vi "Autonomous Independent.vi"() -> ()   [LabVIEW 2013]
doc: "This VI is called when autonomous begins, and will automatically be terminated when autonomous ends. You can carry out timed or sensor driven robot movement independently without needing to return to the caller."
uses:
  Robot Global Data.vi
  OneBall.ctl
  DoubleSolenoidControl.ctl
  ShooterAction.ctl
  TwoBall.ctl
  CollectorEnum.ctl
  RollerStates.ctl
  TankDriveAction.ctl
panel:
  out "Error out 2":errorcluster
  in  "Error in 2":errorcluster
  out "Error out":errorcluster
  in  "Error in":errorcluster
  # "Be sure to right-click and choose Data Operations>>Make Current Value default if you want to save the array values with the VI"
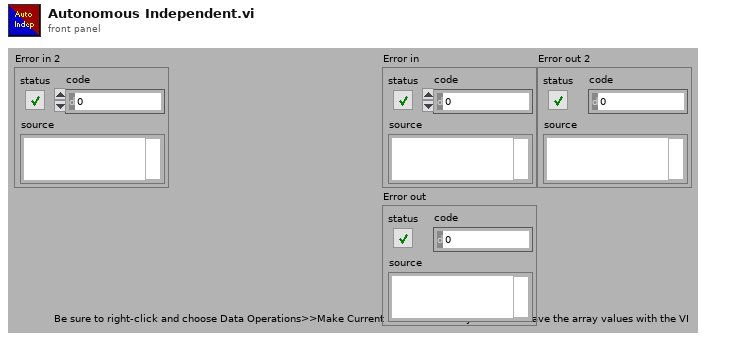
[diagram p1: front panel]
types:
  T1 = typedef "TwoBall.ctl" = enum16{"Init", "Lower Arm", "Spin Roller", "Clapper", "RaiseArmSlightly", "Drive", "Shoot1", "RaiseArmUp", "Shoot2", "Stop"}
  T2 = typedef "OneBall.ctl" = enum16{"Init", "Drive", "Shoot", "CheckGoal", "Stop"}
  T3 = typedef "WPI_JoystickDevRef.ctl" = cluster{"Device":T4}
  T4 = typedef "WPI_JoystickDeviceEnum.ctl" = enum16{"USB 1", "USB 2", "USB 3", "USB 4", "Kinect 1", "Kinect 2"}
  T5 = cluster{"axis 1 (x)":dbl, "axis 2 (y)":dbl, "axis 3 (throttle)":dbl, "axis 4":dbl, "axis 5":dbl, "axis 6":dbl}
  T6 = typedef "DoubleSolenoidControl.ctl" = enum16{"Init", "Out", "In", "Middle"}
  T7 = typedef "CollectorEnum.ctl" = enum16{"Init", "Raise", "Lower", "Stop", "GetStatus"}
  T8 = typedef "TankDriveAction.ctl" = enum16{"Init", "LinearDrive", "SetValue", "Disable"}
  T9 = typedef "RollerStates.ctl" = enum16{"Init", "Off", "Forward", "Reverse"}
  T10 = typedef "ShooterAction.ctl" = enum16{"Init", "Shoot"}
  T11 = typedef "WPI_SolenoidDevRef.ctl" = cluster{"DevStatus":errorcluster, "Solenoid Module":T12, "Forward Solenoid Channel":T13, "Reverse Solenoid Channel":T13}
  T12 = typedef "FPGA_TypedefSolenoidModule.ctl" = enum16{"Solenoid Module 1", "Solenoid Module 2"}
  T13 = typedef "WPI_SolenoidChannel.ctl" = enum8{"Solenoid 1", "Solenoid 2", "Solenoid 3", "Solenoid 4", "Solenoid 5", "Solenoid 6", "Solenoid 7", "Solenoid 8", "Invalid"}
  T14 = typedef "WPI_RelayDevRef.ctl" = cluster{"DevStatus":errorcluster, "Relay Channel":T15, "Digital Module":T16, "Relay Direction":T17}
  T15 = typedef "FPGA_DIORelayChannel.ctl" = enum8{"Relay 1", "Relay 2", "Relay 3", "Relay 4", "Relay 5", "Relay 6", "Relay 7", "Relay 8", "Invalid"}
  T16 = typedef "FPGA_TypedefDigitalModule.ctl" = enum16{"Digital Module 1", "Digital Module 2"}
  T17 = typedef "WPI_RelayDirection.ctl" = enum16{"Both directions", "Forward only", "Reverse only"}
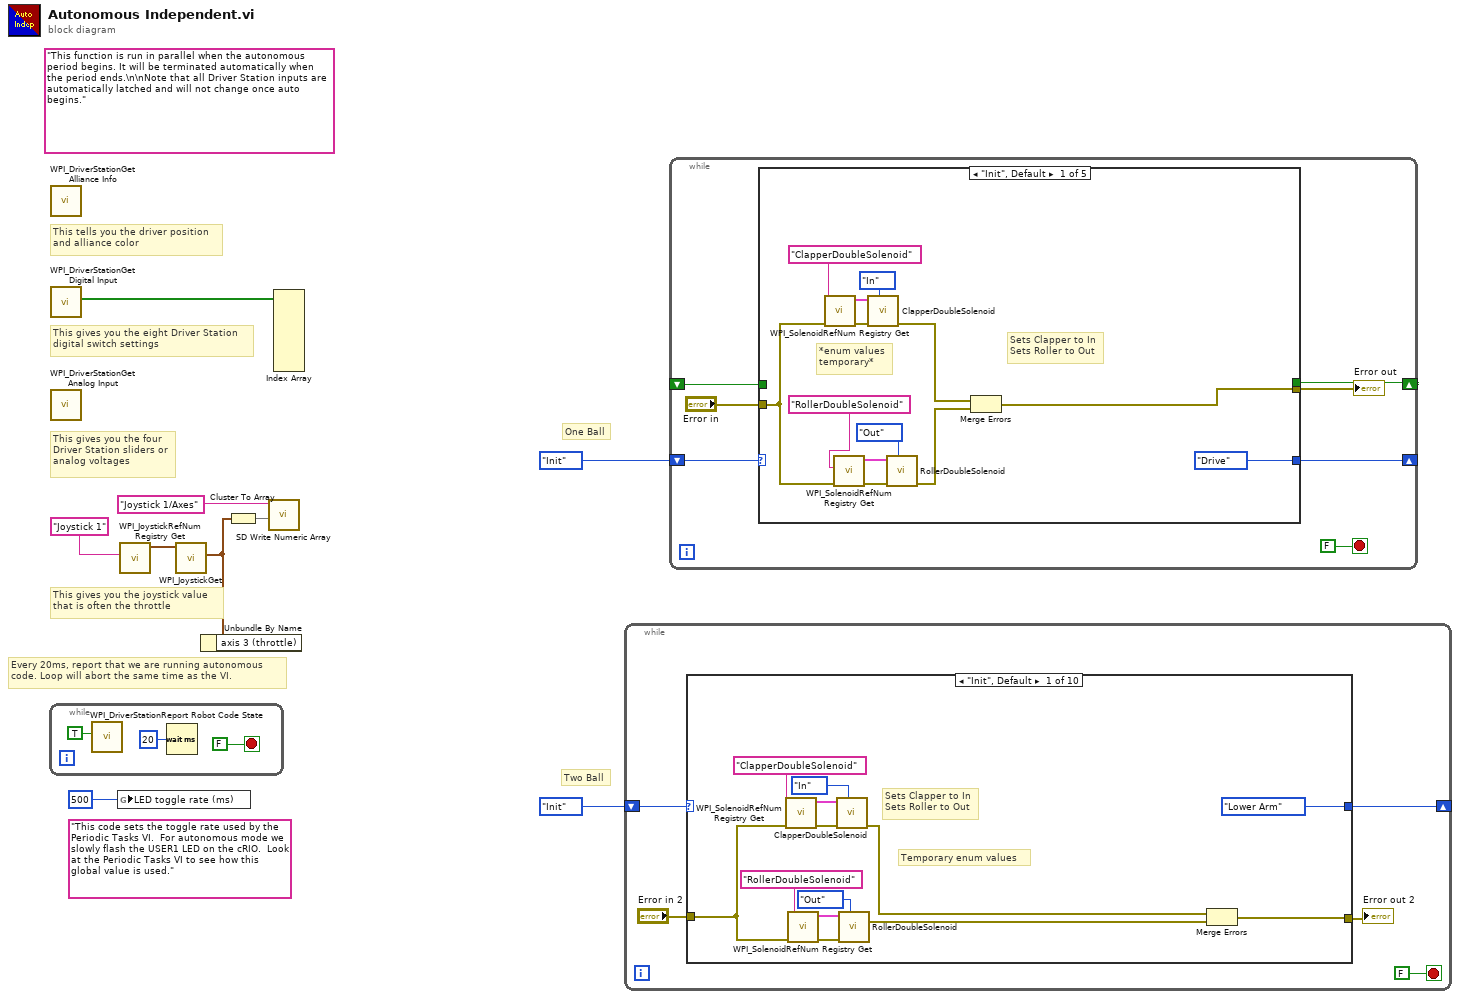
[diagram p0: block diagram]
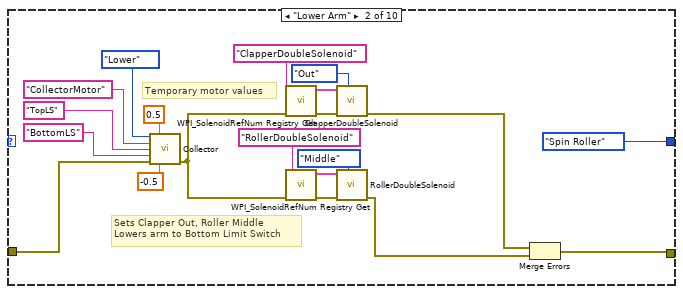
[diagram p2: hidden frame]
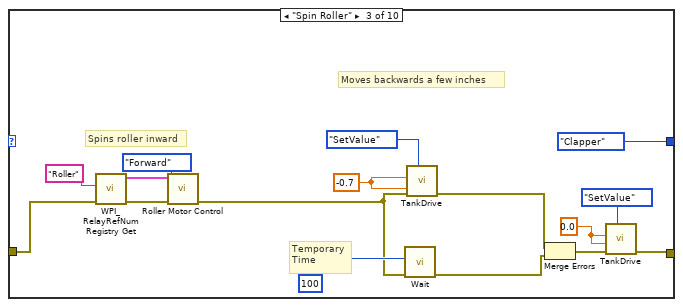
[diagram p3: hidden frame]
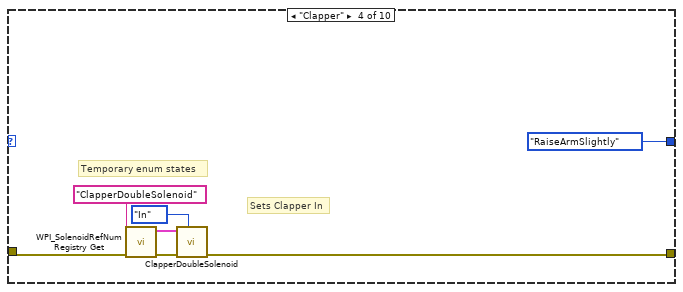
[diagram p4: hidden frame]
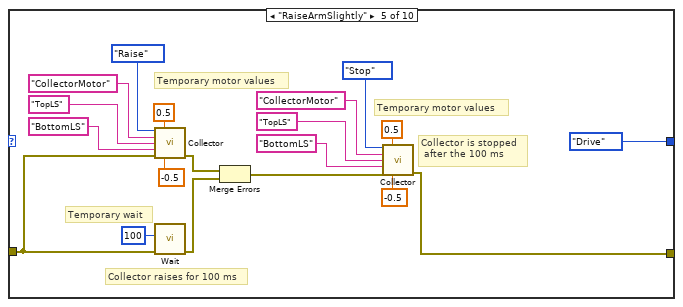
[diagram p5: hidden frame]
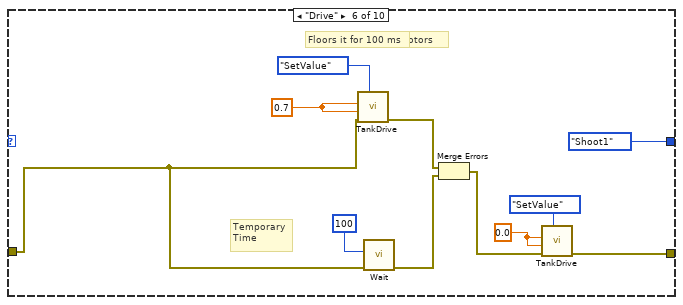
[diagram p6: hidden frame]
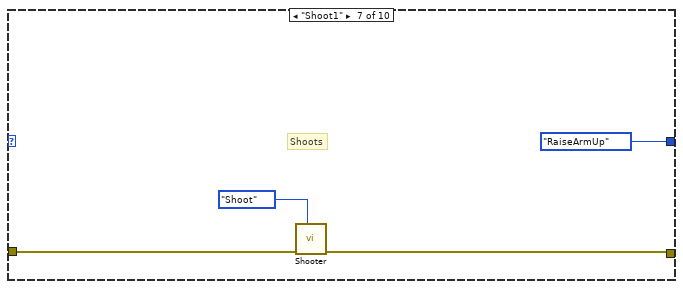
[diagram p7: hidden frame]
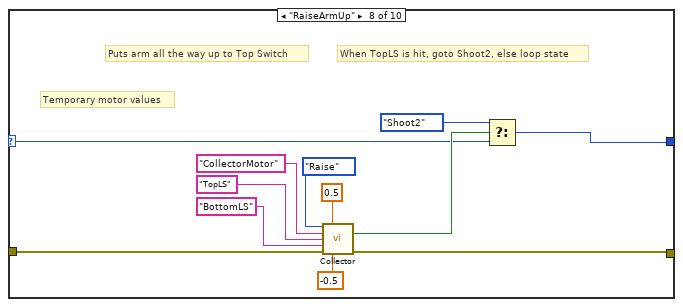
[diagram p8: hidden frame]
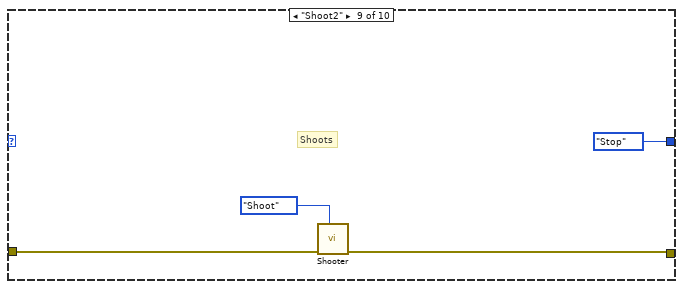
[diagram p9: hidden frame]
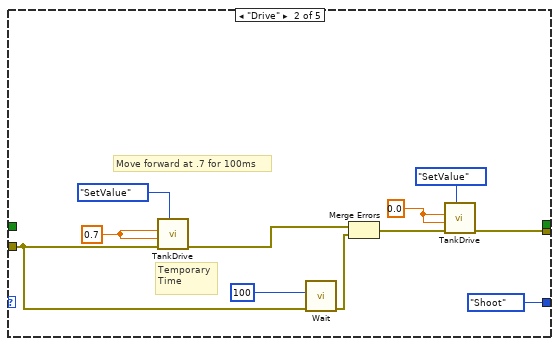
[diagram p11: hidden frame]
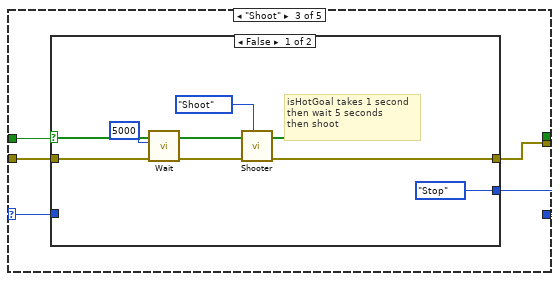
[diagram p12: hidden frame]
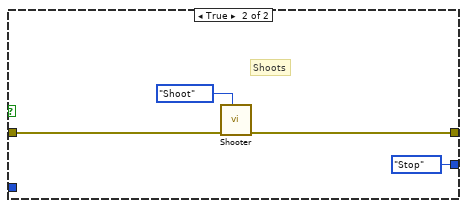
[diagram p13: hidden frame]
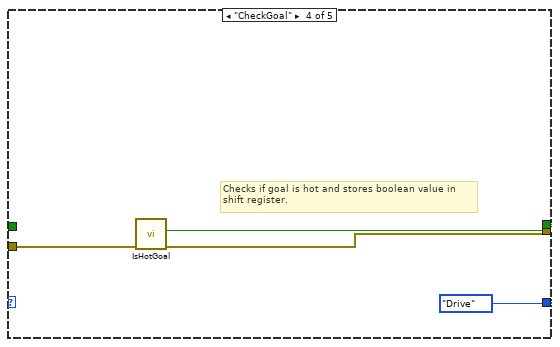
[diagram p14: hidden frame]
diagram:
  (unwired) "This code sets the toggle rate used by the Periodic Tasks VI.  For autonomous mode we slowly flash the USER1 LED on the cRIO.  Look at the Periodic Tasks VI to see how this global value is used."
  (unwired) "This function is run in parallel when the autonomous period begins. It will be terminated automatically when the period ends.\n\nNote that all Driver Station inputs are automatically latched and will not change once auto begins."
  # "Two Ball"
  # "One Ball"
  # "Every 20ms, report that we are running autonomous\ncode. Loop will abort the same time as the VI."
  # "This gives you the joystick value\nthat is often the throttle"
  # "This tells you the driver position\nand alliance color"
  # "This gives you the eight Driver Station\ndigital switch settings"
  # "This gives you the four\nDriver Station sliders or\nanalog voltages"
  n1 = while {
    stop <- FALSE stop-if-true
    n2 = call <vilib>:"WPI_DriverStationReport Robot Code State.vi"("Autonomous"=TRUE) -> ()  [unwired: 10 in, 1 out]
    n3 = Wait (ms)(milliseconds to wait=u32 20) -> ()  [unwired: 1 out]
  }
  n4 = call <vilib>:"WPI_DriverStationGet Alliance Info.vi"() -> ()  [unwired: 12 out]
  n5 = call <vilib>:"WPI_DriverStationGet Digital Input.vi"() -> ("Driver Station Digital Input (1-8)"=w9:bool[])  [unwired: 11 out]
  n6 = call <vilib>:"WPI_DriverStationGet Analog Input.vi"() -> ()  [unwired: 12 out]
  n7 = global write "Robot Global Data.vi" "LED toggle rate (ms)"(u32 500 ("LED ms toggle rate")) -> ()
  n8 = call <vilib>:"WPI_JoystickRefNum Registry Get.vi"("refnum name"="Joystick 1") -> ("JoystickDevRef"=w7:T3)  [unwired: 1 in, 9 out]
  n9 = call <vilib>:"WPI_JoystickGet.vi"("JoystickDevRef"=w7) -> ("Axes"=w3:T5)  [unwired: 1 in, 5 out]
  n10 = Unbundle By Name(w3) -> ()  [unwired: 1 out]
  n11 = Cluster To Array(cluster=w3) -> (array=w5:dbl[])
  n12 = call <vilib>:"SD Write Numeric Array.vi"("Numeric Array"=w5, "Name"="Joystick 1/Axes") -> ()  [unwired: 8 in, 2 out]
  n13 = Index Array(array=w9) -> ()  [unwired: 8 in, 8 out]
  n14 = while {
    shift-right: [w15] -> _
    shift-left: TwoBall."Init" ("Enum") -> [w16]
    stop <- FALSE stop-if-true
    n15 = case shown="\"Init\", Default" w16 {
      selector: w16 -> [_ _ _ _ _ _ _ w108 _ _]
      tunnel: [TwoBall."Lower Arm" ("Enum") TwoBall."Spin Roller" ("Enum") TwoBall."Clapper" ("Enum") TwoBall."RaiseArmSlightly" ("Enum") TwoBall."Drive" ("Enum") TwoBall."Shoot1" ("Enum") TwoBall."RaiseArmUp" ("Enum") w111 TwoBall."Stop" ("Enum") _] -> w15
      tunnel: "Error in 2" -> [w21 w49 w62 w69 w87 w98 w106 w114 w122 w124]
      tunnel: [w18 w36 w53 w68 w75 w95 w105 w113 w121 w124] -> w13
      frame "Init", Default {
        # "Sets Clapper to In\nSets Roller to Out"
        # "Temporary enum values"
        n16 = call <vilib>:"WPI_SolenoidRefNum Registry Get.vi"("error in (no error)"=w21, "refnum name"="ClapperDoubleSolenoid") -> ("error out"=w28:errorcluster, "SolenoidDevRef"=w29:T11)  [unwired: 8 in]
        n17 = call <vilib>:"WPI_SolenoidRefNum Registry Get.vi"("error in (no error)"=w21, "refnum name"="RollerDoubleSolenoid") -> ("error out"=w26:errorcluster, "SolenoidDevRef"=w24:T11)  [unwired: 8 in]
        n18 = call "ClapperDoubleSolenoid.vi"("State"=DoubleSolenoidControl."In", "Error in"=w28, "SolenoidDevRef"=w29) -> ("Error out"=w20:errorcluster)  [unwired: 8 in]
        n19 = call "RollerDoubleSolenoid.vi"("State"=DoubleSolenoidControl."Out", "Error in"=w26, "SolenoidDevRef"=w24) -> ("Error out"=w19:errorcluster)  [unwired: 8 in]
        n20 = Merge Errors(w20, w19) -> (w18:errorcluster)
      }
      frame "Lower Arm" {
        # "Sets Clapper Out, Roller Middle\nLowers arm to Bottom Limit Switch"
        # "Temporary motor values"
        n21 = call "Collector.vi"("CollectorAction"=CollectorEnum."Lower", "Raise"=0.5, "CollectorMotor"="CollectorMotor", "TopLS"="TopLS", "BottomLS"="BottomLS", "Error in"=w49, "Lower"=-0.5) -> ("Error out"=w37:errorcluster)  [unwired: 6 in, 2 out]
        n22 = call <vilib>:"WPI_SolenoidRefNum Registry Get.vi"("error in (no error)"=w37, "refnum name"="ClapperDoubleSolenoid") -> ("error out"=w40:errorcluster, "SolenoidDevRef"=w39:T11)  [unwired: 8 in]
        n23 = call <vilib>:"WPI_SolenoidRefNum Registry Get.vi"("error in (no error)"=w37, "refnum name"="RollerDoubleSolenoid") -> ("error out"=w42:errorcluster, "SolenoidDevRef"=w44:T11)  [unwired: 8 in]
        n24 = call "ClapperDoubleSolenoid.vi"("State"=DoubleSolenoidControl."Out", "Error in"=w40, "SolenoidDevRef"=w39) -> ("Error out"=w35:errorcluster)  [unwired: 8 in]
        n25 = call "RollerDoubleSolenoid.vi"("State"=DoubleSolenoidControl."Middle", "Error in"=w42, "SolenoidDevRef"=w44) -> ("Error out"=w34:errorcluster)  [unwired: 8 in]
        n26 = Merge Errors(w35, w34) -> (w36:errorcluster)
      }
      frame "Spin Roller" {
        w51 = 0.0
        w58 = -0.7
        # "Spins roller inward"
        # "Moves backwards a few inches"
        # "Temporary\nTime"
        n27 = call <vilib>:"WPI_RelayRefNum Registry Get.vi"("error in (no error)"=w62, "refnum name"="Roller") -> ("error out"=w65:errorcluster, "RelayDevRef"=w66:T14)  [unwired: 8 in]
        n28 = call "Roller Motor Control.vi"("Error in"=w65, "RollerState"=RollerStates."Forward", "RelayDevRef"=w66) -> ("Error out"=w54:errorcluster)  [unwired: 8 in]
        n29 = call "Wait.vi"("error in"=w54, "milliseconds to wait"=u32 100) -> ("error out"=w55:errorcluster)  [unwired: 9 in]
        n30 = call "TankDrive.vi"("DriveAction"=TankDriveAction."SetValue", "error in (no error)"=w54, "RightDesired"=w58, "LeftDesired"=w58) -> ("error out"=w56:errorcluster)  [unwired: 7 in]
        n31 = Merge Errors(w56, w55) -> (w60:errorcluster)
        n32 = call "TankDrive.vi"("DriveAction"=TankDriveAction."SetValue", "error in (no error)"=w60, "RightDesired"=w51, "LeftDesired"=w51) -> ("error out"=w53:errorcluster)  [unwired: 7 in]
      }
      frame "Clapper" {
        # "Sets Clapper In"
        # "Temporary enum states"
        n33 = call <vilib>:"WPI_SolenoidRefNum Registry Get.vi"("error in (no error)"=w69, "refnum name"="ClapperDoubleSolenoid") -> ("error out"=w71:errorcluster, "SolenoidDevRef"=w72:T11)  [unwired: 8 in]
        n34 = call "ClapperDoubleSolenoid.vi"("State"=DoubleSolenoidControl."In", "Error in"=w71, "SolenoidDevRef"=w72) -> ("Error out"=w68:errorcluster)  [unwired: 8 in]
      }
      frame "RaiseArmSlightly" {
        # "Collector is stopped\n after the 100 ms"
        # "Collector raises for 100 ms"
        # "Temporary motor values"
        # "Temporary motor values"
        # "Temporary wait"
        n35 = call "Collector.vi"("CollectorAction"=CollectorEnum."Raise", "Raise"=0.5, "CollectorMotor"="CollectorMotor", "TopLS"="TopLS", "BottomLS"="BottomLS", "Error in"=w87, "Lower"=-0.5) -> ("Error out"=w84:errorcluster)  [unwired: 6 in, 2 out]
        n36 = call "Wait.vi"("error in"=w87, "milliseconds to wait"=u32 100) -> ("error out"=w83:errorcluster)  [unwired: 9 in]
        n37 = Merge Errors(w84, w83) -> (w79:errorcluster)
        n38 = call "Collector.vi"("CollectorAction"=CollectorEnum."Stop", "Raise"=0.5, "CollectorMotor"="CollectorMotor", "TopLS"="TopLS", "BottomLS"="BottomLS", "Error in"=w79, "Lower"=-0.5) -> ("Error out"=w75:errorcluster)  [unwired: 6 in, 2 out]
      }
      frame "Drive" {
        w93 = 0.0
        w99 = 0.7 ("RightDesired")
        # "0.7 speed for both motors"
        # "Floors it for 100 ms"
        # "Temporary\nTime"
        n39 = call "TankDrive.vi"("DriveAction"=TankDriveAction."SetValue", "error in (no error)"=w98, "RightDesired"=w99, "LeftDesired"=w99) -> ("error out"=w97:errorcluster)  [unwired: 7 in]
        n40 = call "Wait.vi"("error in"=w98, "milliseconds to wait"=u32 100) -> ("error out"=w100:errorcluster)  [unwired: 9 in]
        n41 = Merge Errors(w97, w100) -> (w101:errorcluster)
        n42 = call "TankDrive.vi"("DriveAction"=TankDriveAction."SetValue", "error in (no error)"=w101, "RightDesired"=w93, "LeftDesired"=w93) -> ("error out"=w95:errorcluster)  [unwired: 7 in]
      }
      frame "Shoot1" {
        # "Shoots"
        n43 = call "Shooter.vi"("Action"=ShooterAction."Shoot", "error in"=w106) -> ("error out"=w105:errorcluster)  [unwired: 9 in]
      }
      frame "RaiseArmUp" {
        # "When TopLS is hit, goto Shoot2, else loop state"
        # "Puts arm all the way up to Top Switch"
        # "Temporary motor values"
        n44 = call "Collector.vi"("CollectorAction"=CollectorEnum."Raise", "Raise"=0.5, "CollectorMotor"="CollectorMotor", "TopLS"="TopLS", "BottomLS"="BottomLS", "Error in"=w114, "Lower"=-0.5) -> ("Upper Triggered?"=w110:bool, "Error out"=w113:errorcluster)  [unwired: 6 in, 1 out]
        n45 = Select(t=TwoBall."Shoot2" ("Enum"), s=w110, f=w108) -> (s? t:f=w111:T1)
      }
      frame "Shoot2" {
        # "Shoots"
        n46 = call "Shooter.vi"("Action"=ShooterAction."Shoot", "error in"=w122) -> ("error out"=w121:errorcluster)  [unwired: 9 in]
      }
      frame "Stop" {
        # "Stop?"
      }
    }
    "Error out 2" <- w13
  }
  n47 = while {
    shift-right: [w128] -> _
    shift-left: OneBall."Init" -> [w127]
    shift-right: [w126] -> _
    shift-left: _ -> [w125]
    stop <- FALSE stop-if-true
    n48 = case shown="\"Init\", Default" w127 {
      selector: w127 -> [_ _ w159 _ _]
      tunnel: [w142 w147 w156 w173 w175] -> w131
      tunnel: "Error in" -> [w134 w150 w157 w174 w175]
      tunnel: [OneBall."Drive" OneBall."Shoot" w160 OneBall."Drive" _] -> w128
      tunnel: [_ _ _ w171 _] -> w126
      tunnel: w125 -> [_ _ w158 _ _]
      frame "Init", Default {
        # "Sets Clapper to In\nSets Roller to Out"
        # "*enum values\ntemporary*"
        n49 = call <vilib>:"WPI_SolenoidRefNum Registry Get.vi"("error in (no error)"=w134, "refnum name"="ClapperDoubleSolenoid") -> ("error out"=w140:errorcluster, "SolenoidDevRef"=w143:T11)  [unwired: 8 in]
        n50 = call <vilib>:"WPI_SolenoidRefNum Registry Get.vi"("error in (no error)"=w134, "refnum name"="RollerDoubleSolenoid") -> ("error out"=w136:errorcluster, "SolenoidDevRef"=w137:T11)  [unwired: 8 in]
        n51 = call "ClapperDoubleSolenoid.vi"("State"=DoubleSolenoidControl."In", "Error in"=w140, "SolenoidDevRef"=w143) -> ("Error out"=w141:errorcluster)  [unwired: 8 in]
        n52 = call "RollerDoubleSolenoid.vi"("State"=DoubleSolenoidControl."Out", "Error in"=w136, "SolenoidDevRef"=w137) -> ("Error out"=w132:errorcluster)  [unwired: 8 in]
        n53 = Merge Errors(w141, w132) -> (w142:errorcluster)
      }
      frame "Drive" {
        w145 = 0.0
        w151 = 0.7 ("RightDesired")
        # "Move forward at .7 for 100ms"
        # "Temporary\nTime"
        n54 = call "TankDrive.vi"("DriveAction"=TankDriveAction."SetValue", "error in (no error)"=w150, "RightDesired"=w151, "LeftDesired"=w151) -> ("error out"=w149:errorcluster)  [unwired: 7 in]
        n55 = call "Wait.vi"("error in"=w150, "milliseconds to wait"=u32 100) -> ("error out"=w152:errorcluster)  [unwired: 9 in]
        n56 = Merge Errors(w149, w152) -> (w155:errorcluster)
        n57 = call "TankDrive.vi"("DriveAction"=TankDriveAction."SetValue", "error in (no error)"=w155, "RightDesired"=w145, "LeftDesired"=w145) -> ("error out"=w147:errorcluster)  [unwired: 7 in]
      }
      frame "Shoot" {
        n58 = case shown="False" w158 {
          tunnel: w159 -> [_ _]
          tunnel: [OneBall."Stop" OneBall."Stop"] -> w160
          tunnel: w157 -> [w165 w169]
          tunnel: [w163 w168] -> w156
          frame False {
            # "isHotGoal takes 1 second\nthen wait 5 seconds\nthen shoot"
            n59 = call "Wait.vi"("error in"=w165, "milliseconds to wait"=u32 5000) -> ("error out"=w164:errorcluster)  [unwired: 9 in]
            n60 = call "Shooter.vi"("Action"=ShooterAction."Shoot", "error in"=w164) -> ("error out"=w163:errorcluster)  [unwired: 9 in]
          }
          frame True {
            # "Shoots"
            n61 = call "Shooter.vi"("Action"=ShooterAction."Shoot", "error in"=w169) -> ("error out"=w168:errorcluster)  [unwired: 9 in]
          }
        }
      }
      frame "CheckGoal" {
        # "Checks if goal is hot and stores boolean value in\nshift register."
        n62 = call "IsHotGoal.vi"("error in"=w174) -> ("error out"=w173:errorcluster, "Hot/Not"=w171:bool)  [unwired: 9 in]
      }
      frame "Stop" {
        # "Stop?"
      }
    }
    "Error out" <- w131
  }
